vi "entry type constant.vi"() -> (0 "map":T1)   [LabVIEW 2024, in "summary manager.lvlib"]
uses:
  summary manager.lvlib
  collection type.ctl
  entry type.ctl
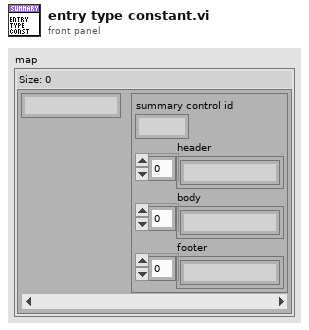
[diagram p1: front panel]
types:
  T1 = typedef "summary manager.lvlib/collection type.ctl" = map{string, T2}
  T2 = typedef "summary manager.lvlib/entry type.ctl" = cluster{"summary control id":i32, "header":string[], "body":string[], "footer":string[]}
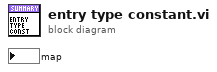
[diagram p0: block diagram]
diagram:
